vi "Write Init acquisition time.vi"(8 "error in (no error)":errorcluster, 10 "Init acquisition time":dbl, 11 "Sync Box in":refnum<class "Sync Box.lvclass">) -> (0 "error out":errorcluster, 3 "Sync Box out":refnum<class "Sync Box.lvclass">)   [LabVIEW 2018, in "Sync Box.lvclass"]
uses:
  Sync Box.lvclass
  Sync Box.lvclass/Sync Box.ctl
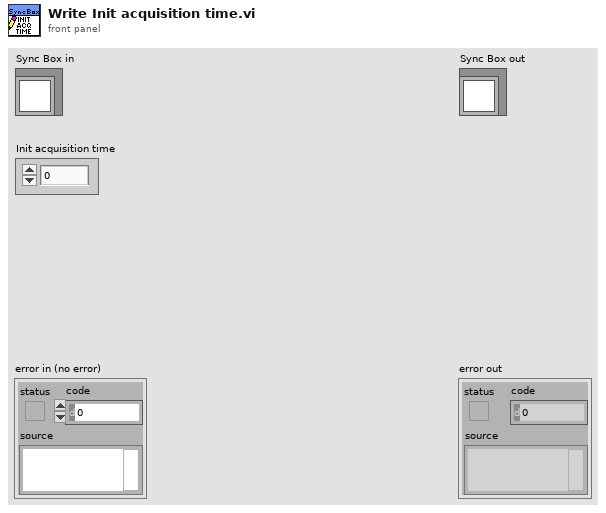
[diagram p1: front panel]
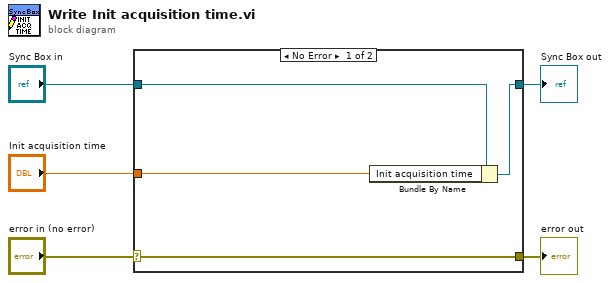
[diagram p0: block diagram]
diagram:
  n1 = case shown="No Error" "error in (no error)" {
    selector: "error in (no error)" -> [w9 w10]
    tunnel: [w9 w10] -> w4
    tunnel: [w7 w11] -> w2
    tunnel: "Sync Box in" -> [w8 w11]
    tunnel: "Init acquisition time" -> [w6 _]
    frame No Error {
      n2 = Bundle By Name(cluster=w8, "Init acquisition time"=w6) -> (w7:refnum<class "Sync Box.lvclass">)
    }
    frame Error {
    }
  }
  "error out" <- w4
  "Sync Box out" <- w2
